vi "Continue Popup.vi"(8 "error in":errorcluster, 11 "Text":string) -> (0 "error out":errorcluster, 3 "Cancel":bool)   [LabVIEW 2015]
uses:
  Lib/Utilities.lvlib
panel:
  in  "Continue":bool=TRUE
  in  "Cancel":bool
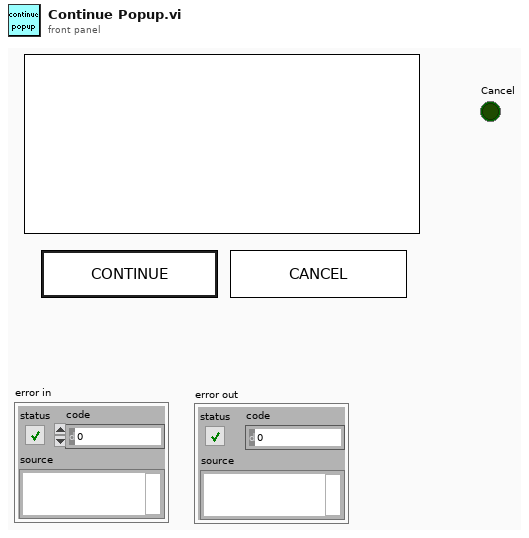
[diagram p1: front panel]
types:
  T1 = enum8{"Enabled", "Disabled", "Disabled and Grayed Out"}
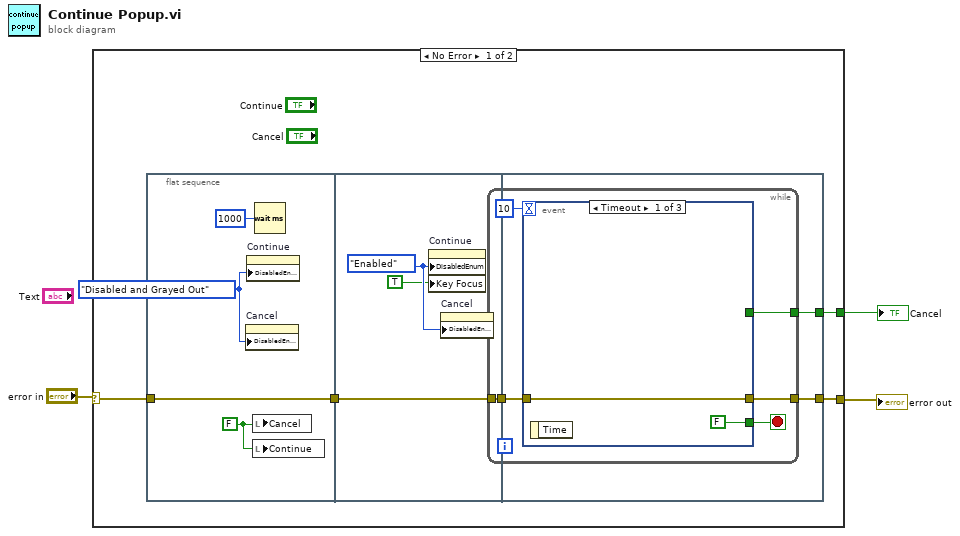
[diagram p0: block diagram]
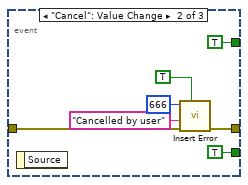
[diagram p2: hidden frame]
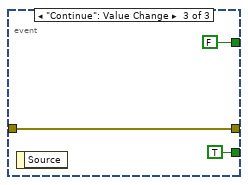
[diagram p3: hidden frame]
diagram:
  n1 = case shown="No Error" "error in" {
    selector: "error in" -> [w8 w36]
    tunnel: [w7 w36] -> w2
    tunnel: [w6 _] -> w1
    frame No Error {
      n2 = flat-sequence {
        tunnel: [w12] -> w5
        tunnel: w8 -> [w12]
        tunnel: w5 -> [w15]
        tunnel: [w15] -> w4
        tunnel: w4 -> [w17]
        tunnel: [w18] -> w7
        tunnel: [w16] -> w6
        frame #0 {
          w9 = T1."Disabled and Grayed Out" ("Disabled")
          w11 = FALSE ("Cancel")
          n3 = property on="Cancel" class="Bool (strict)"("DisabledEnum"=w9) -> ()  [unwired: 2 in, 2 out]
          n4 = property on="Continue" class="Bool (strict)"("DisabledEnum"=w9) -> ()  [unwired: 2 in, 2 out]
          n5 = local write "Cancel"(w11) -> ()
          n6 = local write "Continue"(w11) -> ()
          n7 = Wait (ms)(milliseconds to wait=u32 1000) -> ()  [unwired: 1 out]
        }
        frame #1 {
          w14 = T1."Enabled" ("Disabled")
          n8 = property on="Continue" class="Bool (strict)"("DisabledEnum"=w14, "Key Focus"=TRUE) -> ()  [unwired: 2 in, 2 out]
          n9 = property on="Cancel" class="Bool (strict)"("DisabledEnum"=w14) -> ()  [unwired: 2 in, 2 out]
        }
        frame #2 {
          n10 = while {
            tunnel: [w21] -> w18
            tunnel: w17 -> [w23]
            tunnel: [w19] -> w16
            stop <- w20 stop-if-true
            n11 = event shown="[0] Timeout" {
              selector: _ -> [_ _ _]
              dyn-events: _ -> [_ _ _]
              timeout: 10 -> [_ _ _]
              tunnel: w23 -> [w25 w31 w34]
              tunnel: [w25 w29 w34] -> w21
              tunnel: [FALSE TRUE TRUE] -> w20
              tunnel: [_ TRUE FALSE] -> w19
              event Timeout {
                n12 = event-data() -> ()  [unwired: 1 in, 1 out]
              }
              event "Cancel": Value Change {
                n13 = event-data() -> ()  [unwired: 1 in, 1 out]
                n14 = call "Insert Error.vi"("[error code] (0)"=666, "error description"="Cancelled by user", "error in (no error)"=w31, "error?"=TRUE) -> ("error out"=w29:errorcluster)  [unwired: 6 in]
              }
              event "Continue": Value Change {
                n15 = event-data() -> ()  [unwired: 1 in, 1 out]
              }
            }
          }
        }
      }
    }
    frame Error {
    }
  }
  "error out" <- w2
  "Cancel" <- w1
